vi "MainGUI.vi"() -> ()   [LabVIEW 2018]
uses:
  General/Controls/ScanType.ctl
  General/Controls/Vibratome Parameters.ctl
  General/Controls/Imaging Parameters.ctl
  General/Controls/Scan Direction.ctl
  General/type defines/Alazar parameters.ctl
  Hardware Mfg/AlazarTech SDK/Controls/General Trigger Settings.ctl
  Hardware Mfg/AlazarTech SDK/Controls/Trigger Engine Controls.ctl
  Hardware Mfg/AlazarTech SDK/Controls/Clock Controls.ctl
  Hardware Mfg/AlazarTech SDK/Controls/Alazar Device ID.ctl
  Hardware Mfg/AlazarTech SDK/Controls/Channel Input Controls.ctl
  Hardware Mfg/AlazarTech SDK/Controls/Alazar Acquisition Settings.ctl
  General/Controls/Control cluster.ctl
  General/type defines/file type.ctl
  General/Controls/Optical Parameters.ctl
  General/Controls/Translation Stage Parameters.ctl
  Hardware Mfg/Thorlabs Translation Stages/Controls/Translation Stage Cluster.ctl
  General/Controls/Translation Stage Types.ctl
  General/Controls/Queue Manager Actions.ctl
  General/Controls/MessagePacket.ctl
  General/Controls/QueueNames.ctl
  General/Controls/FGV Actions.ctl
  General/Controls/System Parameters.ctl
  Hardware Mfg/AlazarTech SDK/Controls/Alazar Engine Actions.ctl
  Hardware Mfg/Main Scan Processor Status.vi
  Hardware Mfg/Axsun Laser/Axsun action.ctl
panel:
  in  "Status":string
  in  "Quit":bool
  in  "Acquire":bool
  in  "Control Panel":T1(tab)
  in  "Optical Parameters":T2={"Obj. Focal Length [mm]"=45.0, "Scan Lens EFL[mm]"=59.5, "Tube Lens EFL[mm]"=205.0, "Galvo V Range (+/-)"=10.0, "Galvo Max Half Angle [Deg]"=19.0, "Max Galvo Range[%]"=0.0}
  in  "Galvo HW Parameters":T3={"Analog Out Channel"="GalvoCtrl/ao0,GalvoCtrl/ao1", "Min Voltage"=-10.0, "Max Voltage"=10.0, "Pixel Clock Source"="/GalvoCtrl/PFI0", "Sample Rate"=1000.0, "Line Clock Out Ch"="GalvoCtrl/port0/line0"}
  in  "Imaging Parameter":T4={"Raster Scan Direction"=enum."Uni Directional", "Pixel Dwell Time [Clock Cycles]"=1, "Flyback Time [Clock Cycles]"=200, "XY Center [um]"={"X"=1.0, "Y"=1.0}, "Pixel Step Size [um]"=2.5, "XY Image Size"=enum."2048 x 2048", "Custom"=FALSE, "Custom Size"={"X"=1, "Y"=1}, "Line Averages"=1} {"Line Averages" min=1 max=30 step=1; "Flyback Time [Clock Cycles]" max=1000 step=1; "Pixel Step Size [um]" min=0.0 max=10.0 step=0.01; "Custom Size"."Y" min=1 max=30 step=1; "Custom Size"."X" min=1 max=30 step=1; "XY Center [um]"."Y" min=1.0 max=30.0 step=1.0; "XY Center [um]"."X" min=1.0 max=30.0 step=1.0; "Pixel Dwell Time [Clock Cycles]" max=10 step=1}
  in  "Scan Type":T6
  in  "Alazar parameters":T7={"Trigger Settings"={"General Trigger Settings"={"Trigger Operation"=0, "Coupling ID"=2, "Range ID"=2, "Delay"=0, "Timeout Ticks"=0, "Mode"=1, "Parameter"=1}, "Trigger Engine 1"={"Trigger Engine"=0, "Source"=2, "Slope"=1, "Level"=140}, "Trigger Engine 2"={"Trigger Engine"=1, "Source"=3, "Slope"=1, "Level"=140}}, "Capture Clock"={"Sample Rate"=100, "Decimation"=0, "Source"=2, "Edge"=0}, "Device ID"={"System ID"=1, "Board ID"=1}, "Ch A Input Control"={"Channel"=1, "Coupling"=2, "Range"=10, "Impedance"=2}, "Ch B Input Control"={"Channel"=2, "Coupling"=2, "Range"=10, "Impedance"=2}, "Acq Settings"={"Window Type"=1, "Record Length"=1440, "Footer"=0, "Output Format"=10, "Offset"=0, "Records Per Buffer"=2048, "Samples per record"=2048, "Records Count (Records/Acq)"=2147483647}, "Cluster"={"FFT value magnification"=1000.0, "max queue size (-1, unlimited)"=-1, "File Type"=enum."Tiff", "file path"=path "C:/Users/BoasLab/Documents/Data/Alazar data/B-line/data/test.tif", "#A-lines to save"=2048, "#Z pixels to save"=2048, "ImageDescription"="", "Convert to U16?"=FALSE}} {"Cluster"."FFT value magnification" min=0.0 max=10000.0 step=0.001 format="%.4f"; "Acq Settings"."Window Type" items=["DSP_WINDOW_NONE", "DSP_WINDOW_HANNING", "DSP_WINDOW_HAMMING", "DSP_WINDOW_BLACKMAN", "DSP_WINDOW_BLACKMAN_HARRIS", "DSP_WINDOW_BARTLETT"]; "Acq Settings"."Footer" items=["FOOTER_NONE", "FOOTER_NPT"]; "Acq Settings"."Output Format" items=["FLOAT_AMP2"=10, "FLOAT_LOG"=11]; "Ch B Input Control"."Channel" items=["A"=1, "B"=2, "C"=4, "D"=8]; "Ch B Input Control"."Coupling" items=["AC"=1, "DC"=2]; "Ch B Input Control"."Range" items=["20 mV"=1, "40 mV"=2, "50 mV"=3, "80 mV"=4, "100 mV"=5, "200 mV"=6, "400 mV"=7, "500 mV"=8, "800 mV"=9, "1 V"=10, "1.25 V"=33, "2 V"=11, "4 V"=12, "5 V"=13, "8 V"=14, "10 V"=15, "20 V"=16]; "Ch B Input Control"."Impedance" items=["1 MOhm"=1, "50 Ohm"=2, ""=0]; "Ch A Input Control"."Channel" items=["A"=1, "B"=2, "C"=4, "D"=8]; "Ch A Input Control"."Coupling" items=["AC"=1, "DC"=2]; "Ch A Input Control"."Range" items=["20 mV"=1, "40 mV"=2, "50 mV"=3, "80 mV"=4, "100 mV"=5, "200 mV"=6, "400 mV"=7, "500 mV"=8, "800 mV"=9, "1 V"=10, "1.25 V"=33, "2 V"=11, "4 V"=12, "5 V"=13, "8 V"=14, "10 V"=15, "20 V"=16]; "Ch A Input Control"."Impedance" items=["1 MOhm"=1, "50 Ohm"=2, ""=0]; "Capture Clock"."Edge" items=["Rising", "Falling"]; "Capture Clock"."Source" items=["Internal"=1, "Fast External"=2, "Medium External"=3, "Slow External"=4, "External AC"=5, "External DC"=6, "External 10MHz"=7]; "Trigger Settings"."General Trigger Settings"."Trigger Operation" items=["J", "K", "J OR K", "J AND K", "J XOR K", "J AND NOT K", "NOT J AND K"]; "Trigger Settings"."General Trigger Settings"."Coupling ID" items=["AC"=1, "DC"=2]; "Trigger Settings"."General Trigger Settings"."Range ID" items=["5 V", "1 V", "TTL"]; "Trigger Settings"."Trigger Engine 1"."Trigger Engine" items=["J", "K"]; "Trigger Settings"."Trigger Engine 1"."Source" items=["A", "B", "External", "Disable", "C", "D"]; "Trigger Settings"."Trigger Engine 1"."Slope" items=["Positive"=1, "Negative"=2]; "Trigger Settings"."Trigger Engine 2"."Trigger Engine" items=["J", "K"]; "Trigger Settings"."Trigger Engine 2"."Source" items=["A", "B", "External", "Disable", "C", "D"]; "Trigger Settings"."Trigger Engine 2"."Slope" items=["Positive"=1, "Negative"=2]}
  in  "Vibratome":T16={"Z Bottom [mm]"=0.0, "Pre Cut Dwell [s]"=0.0, "Blade Frequency [RPM]"=0, "Slice Speed [mm/s]"=0.0, "Post Cut Dwell [s]"=0.0, "Ramp Time [s]"=0.0, "Start X [mm]"=0.0, "Start Y [mm]"=0.0, "Slice Length [mm]"=0.0, "Slice Axis"=enum."X Axis", "Controller VISA Ref"="COM4"}
  in  "Mosaic Paramter":T17
  in  "Center Galvos":bool
  in  "path":path=path "C:/Users/BOAS-USER/Documents/Data/0507/human"
  out "time for pre-process":dbl
  out "Error Out":errorcluster
  in  "#pixels to save":i32=200
  in  "start pixel":i32
  in  "Save":bool
  out "elements in display queue":i32
  out "# elements in save queue":i32
  in  "display pixels":i32=500
  in  "FOV: #A-lines":i32=2048
  in  "Init":bool
  in  "Channel":u32(ring)=1 items=["A"=1, "B"=2, "A + B"=3, "C"=4, "A + C"=5, "A + B"=6, "D"=8, "A + D"=9, "B + D"=10, "C + D"=12, "A + B + C + D"=15]
  out "#C-lines":i32=1
  out "# elements in data queue":i32
  in  "Start pixel for display":i32=1
  out "Current Position":cluster{"X":dbl, "Y":dbl}
  in  "Table Stages":T18={"X Stage"={"Position"=0.0, "Is.Enabled?"=FALSE, "Is.Connected?"=FALSE, "Device SN"="45876539", "AccelerationMaximum"=20.0, "VelocityMaximum"=20.0, "Acceleration"=10.0, "Velocity"=10.0, "waitTimeout (ms)"=1000, "Model"=enum."Thorlabs LTS", "Is.Homed?"=FALSE}, "Y Stage"={"Position"=0.0, "Is.Enabled?"=FALSE, "Is.Connected?"=FALSE, "Device SN"="45876539", "AccelerationMaximum"=0.0, "VelocityMaximum"=0.0, "Acceleration"=0.0, "Velocity"=0.0, "waitTimeout (ms)"=0, "Model"=enum."None", "Is.Homed?"=FALSE}, "Z Stage"={"Position"=0.0, "Is.Enabled?"=FALSE, "Is.Connected?"=FALSE, "Device SN"="49876924", "AccelerationMaximum"=8.0, "VelocityMaximum"=3.0, "Acceleration"=4.0, "Velocity"=2.0, "waitTimeout (ms)"=1000, "Model"=enum."Thorlabs MLJ", "Is.Homed?"=FALSE}}
  out "Image":T21(plugin-control)
  out "Control Class ID":u32[](array[numeric])
  out "Label Name":string[][](array[string])
  # "Image Settings"
  # "Optical Settings"
  # "X"
  # "X"
  # "Vibratome Settings"
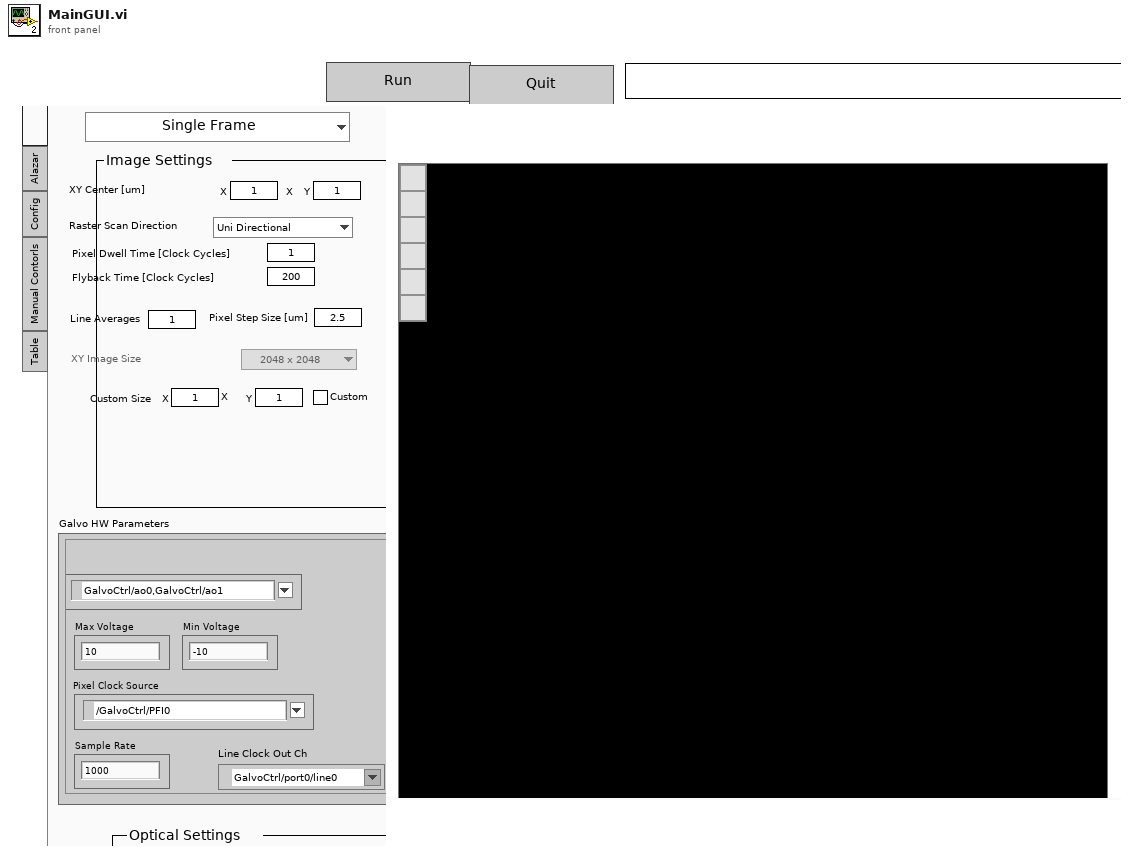
[diagram p1: front panel]
types:
  T1 = enum32{"Galvo", "Alazar", "Config", "Manual Contorls", "Table"}
  T2 = typedef "Optical Parameters.ctl" = cluster{"Obj. Focal Length [mm]":dbl, "Scan Lens EFL[mm]":dbl, "Tube Lens EFL[mm]":dbl, "Galvo V Range (+/-)":dbl, "Galvo Max Half Angle [Deg]":dbl, "Max Galvo Range[%]":dbl}
  T3 = cluster{"Analog Out Channel":tag, "Min Voltage":dbl, "Max Voltage":dbl, "Pixel Clock Source":tag, "Sample Rate":dbl, "Line Clock Out Ch":tag}
  T4 = typedef "Imaging Parameters.ctl" = cluster{"Raster Scan Direction":T5, "Pixel Dwell Time [Clock Cycles]":u16, "Flyback Time [Clock Cycles]":u16, "XY Center [um]":cluster{"X":dbl, "Y":dbl}, "Pixel Step Size [um]":dbl, "XY Image Size":enum16{"32 x 32", "64 x 64", "128 x 128", "256 x 256", "512 x 512", "1024 x 1024", "2048 x 2048"}, "Custom":bool, "Custom Size":cluster{"X":u16, "Y":u16}, "Line Averages":u8}
  T5 = typedef "Scan Direction.ctl" = enum16{"Uni Directional", "Bi Directional", "None"}
  T6 = typedef "ScanType.ctl" = enum16{"Single Frame", "Continuous Frame", "ROI Line", "Vibratome", "Mosaic", "Mosaic + Slice"}
  T7 = typedef "Alazar parameters.ctl" = cluster{"Trigger Settings":cluster{"General Trigger Settings":T8, "Trigger Engine 1":T9, "Trigger Engine 2":T9}, "Capture Clock":T10, "Device ID":T11, "Ch A Input Control":T12, "Ch B Input Control":T12, "Acq Settings":T13, "Cluster":T14}
  T8 = typedef "General Trigger Settings.ctl" = cluster{"Trigger Operation":u32, "Coupling ID":u32, "Range ID":u32, "Delay":u32, "Timeout Ticks":u32, "Mode":u32, "Parameter":u32}
  T9 = typedef "Trigger Engine Controls.ctl" = cluster{"Trigger Engine":u32, "Source":u32, "Slope":u32, "Level":u32}
  T10 = typedef "Clock Controls.ctl" = cluster{"Sample Rate":u32, "Decimation":u32, "Source":u32, "Edge":u32}
  T11 = typedef "Alazar Device ID.ctl" = cluster{"System ID":u32, "Board ID":u32}
  T12 = typedef "Channel Input Controls.ctl" = cluster{"Channel":u8, "Coupling":u32, "Range":u32, "Impedance":u32}
  T13 = typedef "Alazar Acquisition Settings.ctl" = cluster{"Window Type":u32, "Record Length":u32, "Footer":u32, "Output Format":u32, "Offset":u32, "Records Per Buffer":u32, "Samples per record":u32, "Records Count (Records/Acq)":u32}
  T14 = typedef "Control cluster.ctl" = cluster{"FFT value magnification":dbl, "max queue size (-1, unlimited)":i32, "File Type":T15, "file path":path, "#A-lines to save":u32, "#Z pixels to save":u32, "ImageDescription":string, "Convert to U16?":bool}
  T15 = typedef "file type.ctl" = enum16{"text", "Tiff", "binary"}
  T16 = typedef "Vibratome Parameters.ctl" = cluster{"Z Bottom [mm]":dbl, "Pre Cut Dwell [s]":dbl, "Blade Frequency [RPM]":u16, "Slice Speed [mm/s]":dbl, "Post Cut Dwell [s]":dbl, "Ramp Time [s]":dbl, "Start X [mm]":dbl, "Start Y [mm]":dbl, "Slice Length [mm]":dbl, "Slice Axis":enum16{"X Axis", "Y Axis", "Z Axis"}, "Controller VISA Ref":refnum<visa-resource-name>}
  T17 = cluster{"X Axis":cluster{"Start [mm]":dbl, "Steps [pts]":u16, "End [mm]":dbl}, "Y Axis":cluster{"Start [mm]":dbl, "Steps [pts]":u16, "End [mm]":dbl}, "Scan Pattern":enum16{"Uni-directional", "Bi-Directional", "Spiral Out", "Spiral In"}, "Overlap Options":cluster{"Overlap Type":enum16{"No Overlap", "X Only", "Y Only", "X and Y"}, "Percent Overlap":u8, "Justify":enum16{"Start", "Center", "End"}}}
  T18 = typedef "Translation Stage Parameters.ctl" = cluster{"X Stage":T19, "Y Stage":T19, "Z Stage":T19}
  T19 = typedef "Translation Stage Cluster.ctl" = cluster{"Position":dbl, "Is.Enabled?":bool, "Is.Connected?":bool, "Device SN":string, "AccelerationMaximum":dbl, "VelocityMaximum":dbl, "Acceleration":dbl, "Velocity":dbl, "waitTimeout (ms)":i32, "Model":T20, "Is.Homed?":bool}
  T20 = typedef "Translation Stage Types.ctl" = enum16{"None", "Thorlabs LTS", "Thorlabs MLJ"}
  T21 = typedef "IMAQ Image.ctl" = refnum<image>
  T22 = typedef "QueueNames.ctl" = enum16{"Main GUI", "Main Scan Processor", "Main Processing", "Main Saving", "Main Display", "Main Table Stage GUI", "Main Table Stage Proc.", "Scan Engine", "Vibratome GUI", "Vibratome Processor", "Slice Engine"}
  T23 = typedef "Queue Manager Actions.ctl" = enum16{"Init", "Enqueue", "Enqueue All", "Preview Queue", "Dequeue", "Get Status", "Flush Queue", "Flush All Queues", "Release All Queues", "Release Queue", "Enqueue at Opposite End"}
  T24 = typedef "MessagePacket.ctl" = cluster{"Message":string, "Parameter":variant}
  T25 = typedef "Image Type" = u32
  T26 = typedef "Axsun action.ctl" = enum16{"GetSystemStatus", "Clock delay", "GetLaserOnTime", "GetWaveLengthAtSweptTrigger", "Source current ON", "GetSerialNum", "GetControlVersion", "Laser ON", "Laser OFF", "Source current OFF", "Get laser handle", "Start Network Control Interface", "stop", "Create handle"}
  T27 = typedef "FGV Actions.ctl" = enum16{"Init", "Set", "Get", "Clear"}
  T28 = typedef "Alazar Engine Actions.ctl" = enum16{"Init", "Config Clock", "Config Ch", "Config Trig", "Config Non-FFT Acq.", "Non-FFT Acquire", "Load background from Non-FFT buffer", "enable background subtrac", "disable background subtrac", "load background from file", "load background from elsewhere", "start acquire", "background subtraction", "Config Acq.", "Acquire", "UnInit"}
  T29 = enum16{"Set Configuration", "Get Configuration", "Enable Motor", "Disable Motor", "Get Status", "Open Session", "Close Session", "Set Limits", "Get Limits"}
  T30 = typedef "System Parameters.ctl" = cluster{"Optical Parameters":T2, "Vibratome":T16, "Table Stages":T18, "Imaging Parameter":T4, "Galvo HW Parameters":cluster{"Analog Out Channel":tag, "Min Voltage":dbl, "Max Voltage":dbl, "Pixel Clock Source":tag, "Sample Rate":dbl, "Line Clock Out Ch":tag}, "Alazar parameters":T7, "Mosaic Paramter":cluster{"X Axis":cluster{"Start [mm]":dbl, "Steps [pts]":u16, "End [mm]":dbl}, "Y Axis":cluster{"Start [mm]":dbl, "Steps [pts]":u16, "End [mm]":dbl}, "Scan Pattern":enum16{"Uni-directional", "Bi-Directional", "Spiral Out", "Spiral In"}, "Overlap Options":cluster{"Overlap Type":enum16{"No Overlap", "X Only", "Y Only", "X and Y"}, "Percent Overlap":u8, "Justify":enum16{"Start", "Center", "End"}}}}
  T31 = enum16{"32 x 32", "64 x 64", "128 x 128", "256 x 256", "512 x 512", "1024 x 1024", "2048 x 2048"}
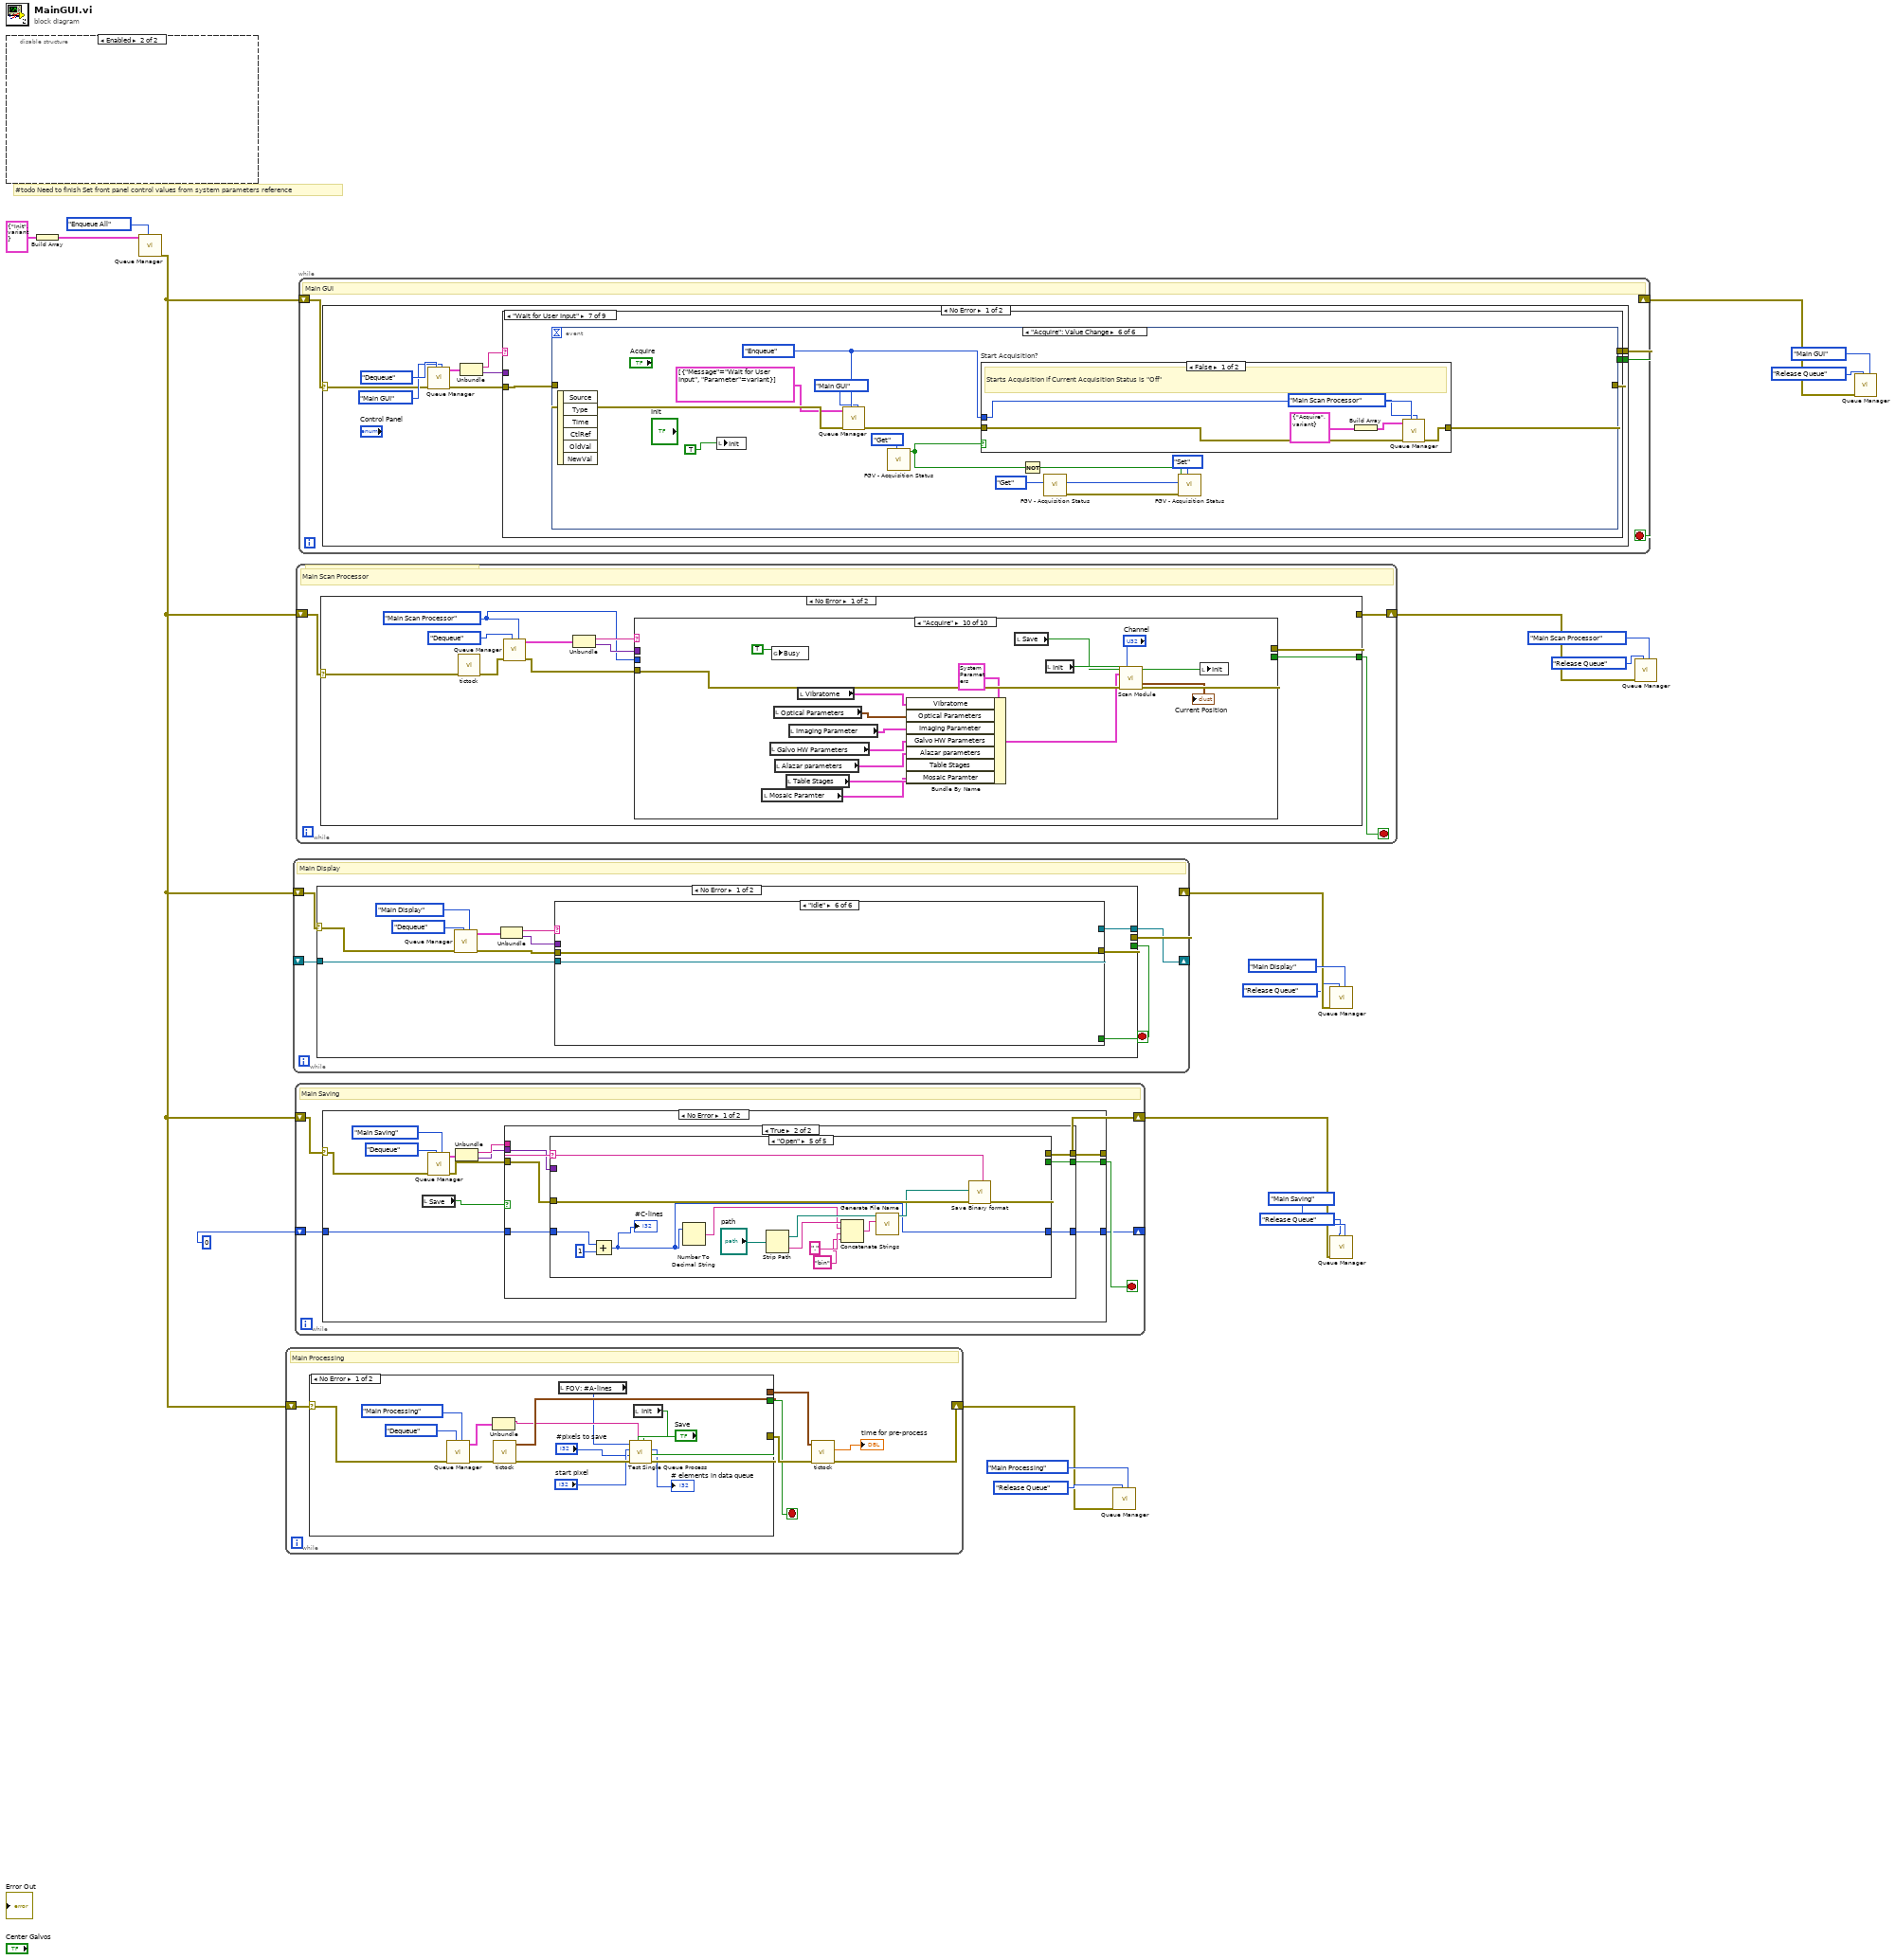
[diagram p0: block diagram]
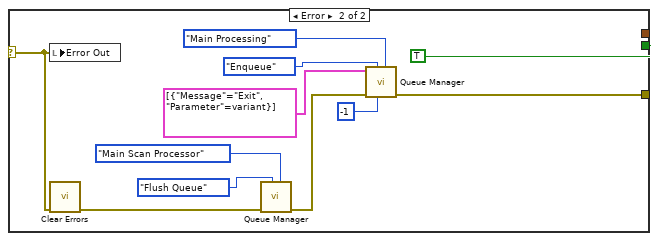
[diagram p2: hidden frame]
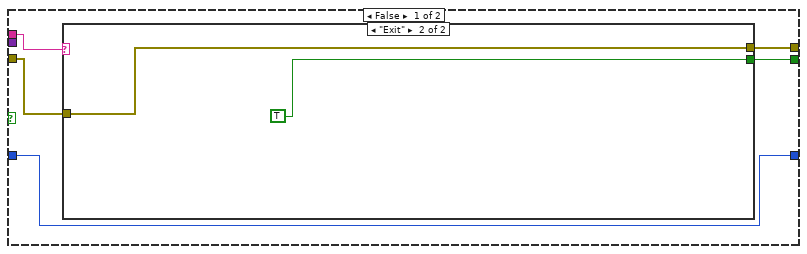
[diagram p3: hidden frame]
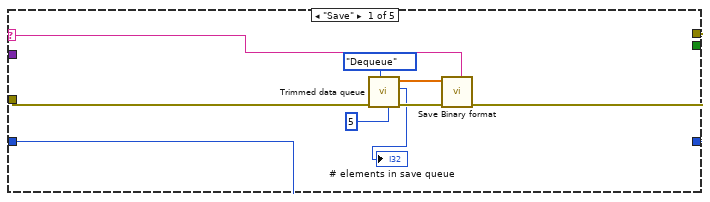
[diagram p5: hidden frame]
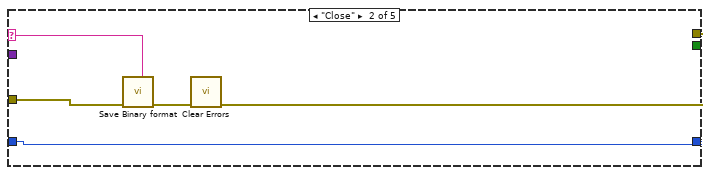
[diagram p6: hidden frame]
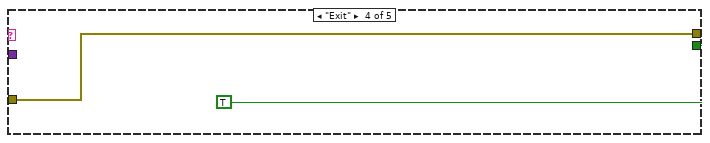
[diagram p8: hidden frame]
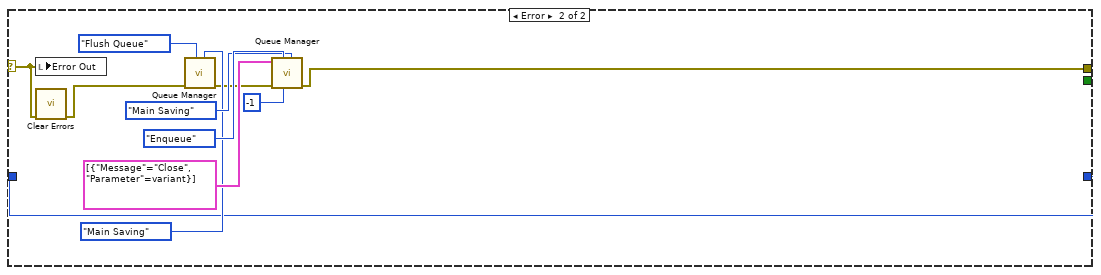
[diagram p9: hidden frame]
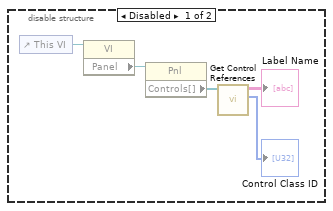
[diagram p10: hidden frame]
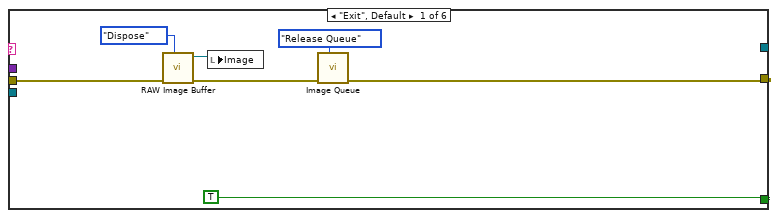
[diagram p11: hidden frame]
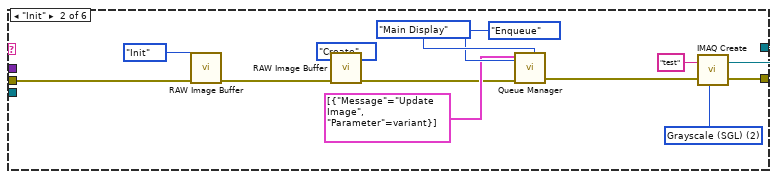
[diagram p12: hidden frame]
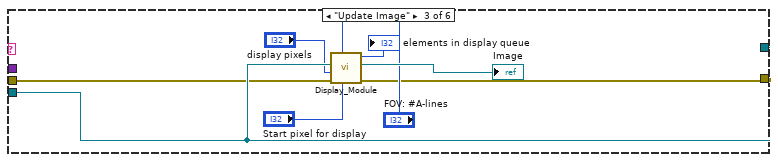
[diagram p13: hidden frame]
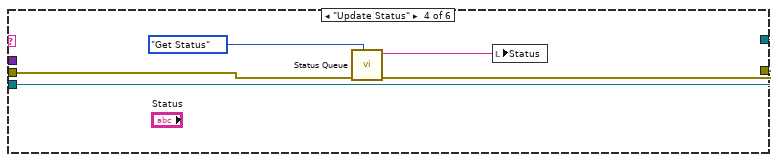
[diagram p14: hidden frame]
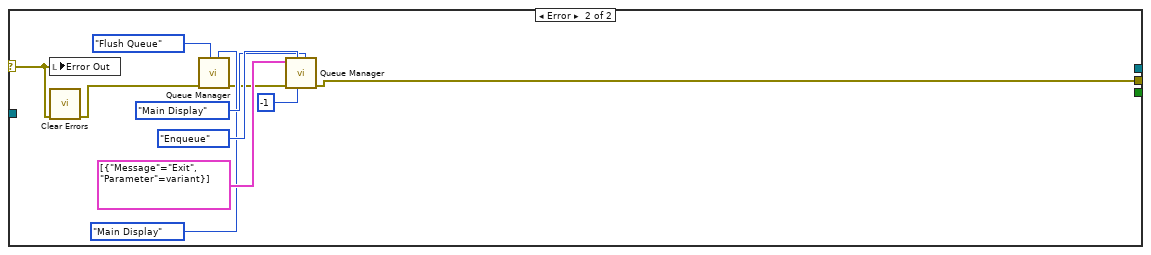
[diagram p16: hidden frame]
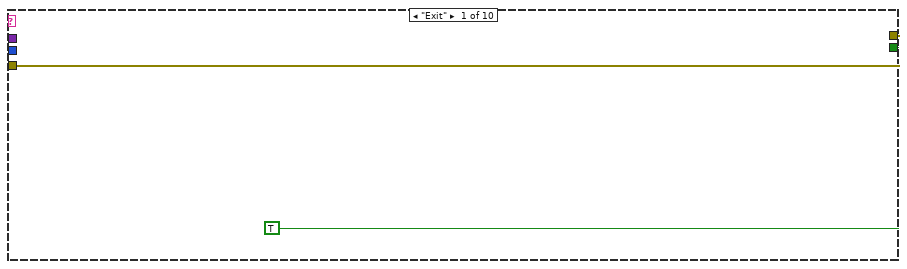
[diagram p17: hidden frame]
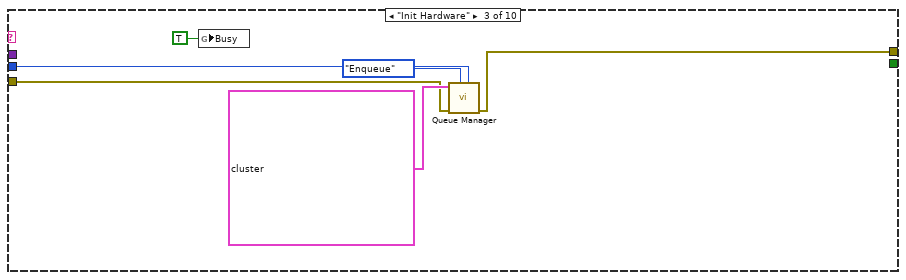
[diagram p19: hidden frame]
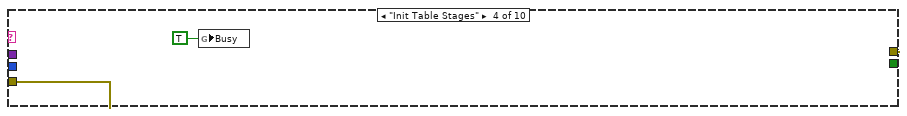
[diagram p20: hidden frame]
diagram:
  # "#todo Add indicator to show connected HW"
  # "#todo Need to finish Set front panel control values from system parameters reference"
  n1 = disable-structure shown="Enabled" {
    frame Disabled {
      n2 = control-ref of="This VI"() -> (w25:refnum<vi>)
      n3 = property class="VI"(reference=w25) -> ("Panel"=w24:refnum<vi>)  [unwired: 1 in, 2 out]
      n4 = property class="Pnl"(reference=w24) -> ("Controls[]"=w23:refnum<vi>[])  [unwired: 1 in, 2 out]
      n5 = call "Get Control References.vi"("Control References"=w23) -> ("Control Class ID"=→"Control Class ID":u32[], "Label Name"=→"Label Name":string[][])  [unwired: 8 in, 1 out]
    }
    frame Enabled {
    }
  }
  n6 = Build Array(T24 {"Message"="Init", "Parameter"=variant} ("Message Packet [In]")) -> (w18:T24[])
  n7 = call "Queue Manager.vi"("Action"=Queue_Manager_Actions."Enqueue All", "Message Packet Array"=w18) -> ("Error Out"=w2:errorcluster)  [unwired: 5 in, 4 out]
  n8 = while "Main Data Processing" {
    shift-right: [w30] -> w3
    shift-left: w2 -> [w28]
    stop <- w26 stop-if-true
    # "Main Processing"
    n9 = case shown="No Error" w28 {
      selector: w28 -> [w42 w54]
      tunnel: [w40 w53] -> w31
      tunnel: [w43 _] -> w29
      tunnel: [w39 TRUE ("Exit?")] -> w26
      frame No Error {
        n10 = call "Queue Manager.vi"("Queue Name"=QueueNames."Main Processing", "Action"=Queue_Manager_Actions."Dequeue", "Error In"=w42) -> ("Error Out"=w44:errorcluster, "Message Packet [Out]"=w45:T24)  [unwired: 4 in, 3 out]
        n11 = Unbundle(w45) -> ("Message"=w37:string)  [unwired: 1 out]
        n12 = call "tictock.vi"("error in (no error)"=w44) -> ("error out"=w41:errorcluster, "seconds since 1Jan1904"=w43:timestamp)  [unwired: 8 in, 1 out]
        n13 = local read "FOV: #A-lines"() -> (w36:i32)
        n14 = local read "Init"() -> (w32:bool)
        n15 = call "Test Single Queue Process.vi"("Init?"=w32, "Action"=w37, "Save"="Save", "error in"=w41, "#pixels to save"="#pixels to save", "start pixel"="start pixel", "#A-lines per B-line"=w36) -> ("Error Out"=w40:errorcluster, "Exit?"=w39:bool, "# elements in data queue"=→"# elements in data queue":i32)  [unwired: 2 in]
      }
      frame Error {
        n16 = local write "Error Out"(w54) -> ()
        n17 = call <vilib>:"Clear Errors.vi"("error in (no error)"=w54) -> ("error out"=w50:errorcluster)  [unwired: 5 in, 1 out]
        n18 = call "Queue Manager.vi"("Queue Name"=QueueNames."Main Scan Processor", "Action"=Queue_Manager_Actions."Flush Queue", "Error In"=w50) -> ("Error Out"=w49:errorcluster)  [unwired: 4 in, 4 out]
        n19 = call "Queue Manager.vi"("Queue Name"=QueueNames."Main Processing", "timeout in ms (-1)"=-1, "Action"=Queue_Manager_Actions."Enqueue", "Error In"=w49, "Message Packet Array"=T24[] [{"Message"="Exit", "Parameter"=variant}] ("Message Packet [In]")) -> ("Error Out"=w53:errorcluster)  [unwired: 2 in, 4 out]
      }
    }
    n20 = call "tictock.vi"("error in (no error)"=w31, "seconds since 1Jan1904 2"=w29) -> ("error out"=w30:errorcluster, "Numeric"=→"time for pre-process":dbl)  [unwired: 7 in, 1 out]
  }
  n21 = while {
    shift-right: [w63] -> w10
    shift-left: w2 -> [w59]
    shift-right: [w61] -> _
    shift-left: _ -> [w60]
    stop <- w62 stop-if-true
    # "Main Display"
    n22 = case shown="No Error" w59 {
      selector: w59 -> [w64 w117]
      tunnel: [w68 w116] -> w63
      tunnel: [w67 _] -> w62
      tunnel: [w66 _] -> w61
      tunnel: w60 -> [w65 _]
      frame No Error {
        n23 = call "Queue Manager.vi"("Queue Name"=QueueNames."Main Display", "Action"=Queue_Manager_Actions."Dequeue", "Error In"=w64) -> ("Error Out"=w72:errorcluster, "Message Packet [Out]"=w71:T24)  [unwired: 4 in, 3 out]
        n24 = Unbundle(w71) -> ("Message"=w70:string, "Parameter"=w69:variant)
        n25 = case shown="\"Idle\"" w70 {
          tunnel: w72 -> [w79 w94 w95 w107 w109 w111]
          tunnel: w69 -> [_ _ _ _ _ _]
          tunnel: [w77 w82 w96 w106 w109 w111] -> w68
          tunnel: [TRUE _ _ _ _ _] -> w67
          tunnel: [_ w88 w102 w103 w108 w110] -> w66
          tunnel: w65 -> [_ _ w102 w103 w108 w110]
          frame "Exit", Default {
            n26 = call "RAW Image Buffer.vi"("Actions"=enum16{"Init", "Create", "Get", "Dispose"}."Dispose", "Error In"=w79) -> ("Error Out"=w78:errorcluster, "Image Out"=w75:T21)  [unwired: 8 in]
            n27 = local write "Image"(w75) -> ()
            n28 = call "Image Queue.vi"("Action"=Queue_Manager_Actions."Release Queue", "Error In"=w78) -> ("Error Out"=w77:errorcluster)  [unwired: 8 in, 1 out]
          }
          frame "Init" {
            w89 = T25 2 items=["Grayscale (U8)", "Grayscale (I16)", "Grayscale (SGL)", "Complex (CSG)", "RGB (U32)", "HSL (U32)", "RGB (U64)", "Grayscale (U16)"] ("Image Type")
            n29 = call "RAW Image Buffer.vi"("Actions"=enum16{"Init", "Create", "Get", "Dispose"}."Init", "Error In"=w94) -> ("Error Out"=w93:errorcluster)  [unwired: 8 in, 1 out]
            n30 = call "RAW Image Buffer.vi"("Actions"=enum16{"Init", "Create", "Get", "Dispose"}."Create", "Error In"=w93) -> ("Error Out"=w84:errorcluster)  [unwired: 8 in, 1 out]
            n31 = call "Queue Manager.vi"("Queue Name"=QueueNames."Main Display", "Action"=Queue_Manager_Actions."Enqueue", "Error In"=w84, "Message Packet Array"=T24[] [{"Message"="Update Image", "Parameter"=variant}]) -> ("Error Out"=w83:errorcluster)  [unwired: 3 in, 4 out]
            n32 = call "IMAQ Create"("Image Name"="test", "Image Type"=w89, "error in (no error)"=w83) -> ("New Image"=w88:T21, "error out"=w82:errorcluster)  [unwired: 2 in]
          }
          frame "Update Image" {
            n33 = call "Display_Module.vi"("Start pixel for display"="Start pixel for display", "FOV: #A-lines"="FOV: #A-lines", "error in"=w95, "Total pixels to display"="display pixels", "Source in"=w102) -> ("error out"=w96:errorcluster, "Image"=→"Image":T21, "elements in display queue"=→"elements in display queue":i32)  [unwired: 4 in]
          }
          frame "Update Status" {
            n34 = call "Status Queue.vi"("Action"=Queue_Manager_Actions."Get Status", "Error In"=w107) -> ("Error Out"=w106:errorcluster, "Status Message [Out]"=w104:string)  [unwired: 8 in]
            n35 = local write "Status"(w104) -> ()
          }
          frame "Update Line Profile" {
          }
          frame "Idle" {
          }
        }
      }
      frame Error {
        n36 = local write "Error Out"(w117) -> ()
        n37 = call <vilib>:"Clear Errors.vi"("error in (no error)"=w117) -> ("error out"=w113:errorcluster)  [unwired: 5 in, 1 out]
        n38 = call "Queue Manager.vi"("Queue Name"=QueueNames."Main Display", "Action"=Queue_Manager_Actions."Flush Queue", "Error In"=w113) -> ("Error Out"=w112:errorcluster)  [unwired: 4 in, 4 out]
        n39 = call "Queue Manager.vi"("Queue Name"=QueueNames."Main Display", "timeout in ms (-1)"=-1, "Action"=Queue_Manager_Actions."Enqueue", "Error In"=w112, "Message Packet Array"=T24[] [{"Message"="Exit", "Parameter"=variant}] ("Message Packet [In]")) -> ("Error Out"=w116:errorcluster)  [unwired: 2 in, 4 out]
      }
    }
  }
  n40 = while {
    shift-right: [w126] -> w6
    shift-left: w2 -> [w124]
    shift-right: [w123] -> _
    shift-left: 0 -> [w122]
    stop <- w125 stop-if-true
    # "Main Saving"
    n41 = case shown="No Error" w124 {
      selector: w124 -> [w136 w192]
      tunnel: [w138 w191] -> w126
      tunnel: [w137 _] -> w125
      tunnel: [w135 w186] -> w123
      tunnel: w122 -> [w134 w186]
      frame No Error {
        n42 = local read "Save"() -> (w133:bool)
        n43 = call "Queue Manager.vi"("Queue Name"=QueueNames."Main Saving", "Action"=Queue_Manager_Actions."Dequeue", "Error In"=w136) -> ("Error Out"=w127:errorcluster, "Message Packet [Out]"=w132:T24)  [unwired: 4 in, 3 out]
        n44 = Unbundle(w132) -> ("Message"=w129:string, "Parameter"=w128:variant)
        n45 = case shown="True" w133 {
          tunnel: [w142 w153] -> w138
          tunnel: [w139 w152] -> w137
          tunnel: [w140 w151] -> w135
          tunnel: w134 -> [w140 w150]
          tunnel: w129 -> [w141 w149]
          tunnel: w128 -> [_ w148]
          tunnel: w127 -> [w143 w147]
          frame False {
            n46 = case shown="\"Exit\"" w141 {
              tunnel: [w144 w145] -> w142
              tunnel: w143 -> [w144 w145]
              tunnel: [_ TRUE] -> w139
              frame "Init", Default {
              }
              frame "Exit" {
              }
            }
          }
          frame True {
            n47 = case shown="\"Open\"" w149 {
              selector: w149 -> [w161 w166 _ _ w184]
              tunnel: [w159 w163 w169 w170 w175] -> w153
              tunnel: w148 -> [_ _ _ _ _]
              tunnel: w147 -> [w162 w167 w169 w170 w185]
              tunnel: [_ _ _ TRUE _] -> w152
              tunnel: [w160 w164 w168 _ w173] -> w151
              tunnel: w150 -> [w160 w164 w168 _ w172]
              frame "Save" {
                n48 = call "Trimmed data queue.vi"("timeout in ms (-1)"=5, "Action"=Queue_Manager_Actions."Dequeue", "error in (no error)"=w162) -> ("error out"=w157:errorcluster, "# elements in queue"=→"# elements in save queue":i32, "data out"=w158:sgl[])  [unwired: 5 in, 1 out]
                n49 = call "Save Binary format.vi"("action"=w161, "error in"=w157, "data in"=w158) -> ("error out"=w159:errorcluster)  [unwired: 8 in]
              }
              frame "Close" {
                n50 = call "Save Binary format.vi"("action"=w166, "error in"=w167) -> ("error out"=w165:errorcluster)  [unwired: 9 in]
                n51 = call <vilib>:"Clear Errors.vi"("error in (no error)"=w165) -> ("error out"=w163:errorcluster)  [unwired: 5 in, 1 out]
              }
              frame "Init", Default {
              }
              frame "Exit" {
              }
              frame "Open" {
                n52 = Add(x=w172, y=1) -> (x+y=w173:i32)
                "#C-lines" <- w173
                n53 = Number To Decimal String(number=w173) -> (decimal integer string=w178:string)  [unwired: 1 in]
                n54 = Strip Path(path="path") -> (stripped path=w182:path, name=w183:string)
                n55 = Concatenate Strings(w183, w178, "." ("string"), "bin" ("string")) -> (w181:string)
                n56 = call "Generate File Name.vi"("name or relative path"=w181, "base path"=w182) -> ("appended path"=w180:path)  [unwired: 9 in]
                n57 = call "Save Binary format.vi"("action"=w184, "error in"=w185, "file path (use dialog)"=w180) -> ("error out"=w175:errorcluster)  [unwired: 8 in]
              }
            }
          }
        }
      }
      frame Error {
        n58 = local write "Error Out"(w192) -> ()
        n59 = call <vilib>:"Clear Errors.vi"("error in (no error)"=w192) -> ("error out"=w188:errorcluster)  [unwired: 5 in, 1 out]
        n60 = call "Queue Manager.vi"("Queue Name"=QueueNames."Main Saving", "Action"=Queue_Manager_Actions."Flush Queue", "Error In"=w188) -> ("Error Out"=w187:errorcluster)  [unwired: 4 in, 4 out]
        n61 = call "Queue Manager.vi"("Queue Name"=QueueNames."Main Saving", "timeout in ms (-1)"=-1, "Action"=Queue_Manager_Actions."Enqueue", "Error In"=w187, "Message Packet Array"=T24[] [{"Message"="Close", "Parameter"=variant}] ("Message Packet [In]")) -> ("Error Out"=w191:errorcluster)  [unwired: 2 in, 4 out]
      }
    }
  }
  n62 = while {
    shift-right: [w198] -> w12
    shift-left: w2 -> [w197]
    stop <- w199 stop-if-true
    # "Main Scan Processor"
    n63 = case shown="No Error" w197 {
      selector: w197 -> [w202 w284]
      tunnel: [w205 _] -> w199
      tunnel: [w200 w279] -> w198
      frame No Error {
        w204 = QueueNames."Main Scan Processor" ("Queue Name")
        n64 = call "tictock.vi"("error in (no error)"=w202) -> ("error out"=w203:errorcluster)  [unwired: 8 in, 2 out]
        n65 = call "Queue Manager.vi"("Queue Name"=w204, "Action"=Queue_Manager_Actions."Dequeue", "Error In"=w203) -> ("Error Out"=w201:errorcluster, "Message Packet [Out]"=w208:T24)  [unwired: 4 in, 3 out]
        n66 = Unbundle(w208) -> ("Message"=w207:string, "Parameter"=w206:variant)
        n67 = case shown="\"Acquire\"" w207 {
          tunnel: w206 -> [_ _ _ _ _ _ _ _ _ _]
          tunnel: [w210 w212 w218 w219 w221 w223 w242 w246 w256 w273] -> w200
          tunnel: [TRUE _ _ _ _ _ _ _ _ _] -> w205
          tunnel: w204 -> [_ _ w217 _ _ _ _ _ _ _]
          tunnel: w201 -> [w210 w212 w213 w219 w221 w222 w237 w245 w256 w270]
          frame "Exit" {
          }
          frame "Init" {
          }
          frame "Init Hardware" {
            n68 = global write "Main Scan Processor Status.vi" "Busy"(TRUE ("Busy")) -> ()
            n69 = call "Queue Manager.vi"("Queue Name"=w217, "Action"=Queue_Manager_Actions."Enqueue", "Error In"=w213, "Message Packet Array"=T24[] [{"Message"="Init Table Stages", "Parameter"=variant}, {"Message"="Init DAQ", "Parameter"=variant}, {"Message"="Init Vibratome", "Parameter"=variant}, {"Message"="Idle", "Parameter"=variant}, {"Message"="Init Laser", "Parameter"=variant}, {"Message"="Init Alazar", "Parameter"=variant}, {"Message"="Init Table Stages", "Parameter"=variant}]) -> ("Error Out"=w218:errorcluster)  [unwired: 3 in, 4 out]
          }
          frame "Init Table Stages" {
            n70 = global write "Main Scan Processor Status.vi" "Busy"(TRUE ("Busy")) -> ()
          }
          frame "Init DAQ" {
          }
          frame "Init Laser" {
            n71 = disable-structure shown="Disabled" {
              disable-tunnel: w222 -> [w225 _]
              disable-tunnel: [w224 _] -> w223
              frame Disabled {
                n72 = call "Axsun module.vi"("Action"=Axsun_action."Create handle", "error in (no error)"=w225) -> ("error out"=w235:errorcluster)  [unwired: 8 in, 1 out]
                n73 = call "Axsun module.vi"("Action"=Axsun_action."GetControlVersion", "error in (no error)"=w235) -> ("error out"=w234:errorcluster)  [unwired: 8 in, 1 out]
                n74 = call "Axsun module.vi"("Action"=Axsun_action."Start Network Control Interface", "error in (no error)"=w234) -> ("error out"=w233:errorcluster)  [unwired: 8 in, 1 out]
                n75 = call "Axsun module.vi"("Action"=Axsun_action."Get laser handle", "error in (no error)"=w233) -> ("error out"=w232:errorcluster)  [unwired: 8 in, 1 out]
                n76 = call "Axsun module.vi"("Action"=Axsun_action."GetSerialNum", "error in (no error)"=w232) -> ("error out"=w231:errorcluster)  [unwired: 8 in, 1 out]
                n77 = call "Axsun module.vi"("Action"=Axsun_action."GetSystemStatus", "error in (no error)"=w231) -> ("error out"=w224:errorcluster)  [unwired: 8 in, 1 out]
              }
              frame Enabled {
              }
            }
          }
          frame "Init Alazar" {
            n78 = call "System Parameters - FGV.vi"("Actions"=FGV_Actions."Get", "Error In"=w237) -> ("Error Out"=w240:errorcluster, "System Parameters"=w239:T30)  [unwired: 8 in]
            n79 = Unbundle By Name(w239) -> ("Alazar parameters"=w238:T7)
            n80 = Unbundle By Name(w238) -> ("Device ID"=w243:T11)
            n81 = call "AlazarEngine.vi"("Action"=Alazar_Engine_Actions."Init", "error in (no error)"=w240, "Device ID"=w243) -> ("error out"=w242:errorcluster)  [unwired: 6 in, 2 out]
          }
          frame "Init Vibratome" {
            n82 = disable-structure shown="Disabled" {
              disable-tunnel: w245 -> [w252 _]
              disable-tunnel: [w251 _] -> w246
              frame Disabled {
                n83 = call "System Parameters - FGV.vi"("Actions"=FGV_Actions."Get") -> ("System Parameters"=w249:T30)  [unwired: 9 in, 1 out]
                n84 = Unbundle By Name(w249) -> ("Vibratome.Controller VISA Ref"=w248:refnum<visa-resource-name>)
                n85 = call "MCDC3006 Module.vi"("Actions"=T29."Open Session", "Error In"=w252, "VISA resource name"=w248) -> ("Error Out"=w254:errorcluster)  [unwired: 4 in, 4 out]
                n86 = call "MCDC3006 Module.vi"("Actions"=T29."Enable Motor", "Error In"=w254) -> ("Error Out"=w251:errorcluster)  [unwired: 5 in, 4 out]
              }
              frame Enabled {
              }
            }
            n87 = global write "Main Scan Processor Status.vi" "Busy"(TRUE ("Busy")) -> ()
          }
          frame "Idle", Default {
            n88 = global write "Main Scan Processor Status.vi" "Busy"(FALSE ("Busy")) -> ()
          }
          frame "Acquire" {
            n89 = local read "Mosaic Paramter"() -> (w260:T17)
            n90 = local read "Galvo HW Parameters"() -> (w265:T3)
            n91 = global write "Main Scan Processor Status.vi" "Busy"(TRUE ("Busy")) -> ()
            n92 = local read "Optical Parameters"() -> (w267:T2)
            n93 = local read "Alazar parameters"() -> (w264:T7)
            n94 = local read "Table Stages"() -> (w263:T18)
            n95 = local read "Imaging Parameter"() -> (w266:T4)
            n96 = local read "Vibratome"() -> (w268:T16)
            n97 = Bundle By Name(cluster=T30 {"Optical Parameters"={"Obj. Focal Length [mm]"=0.0, "Scan Lens EFL[mm]"=0.0, "Tube Lens EFL[mm]"=0.0, "Galvo V Range (+/-)"=0.0, "Galvo Max Half Angle [Deg]"=0.0, "Max Galvo Range[%]"=0.0}, "Vibratome"={"Z Bottom [mm]"=0.0, "Pre Cut Dwell [s]"=0.0, "Blade Frequency [RPM]"=0, "Slice Speed [mm/s]"=0.0, "Post Cut Dwell [s]"=0.0, "Ramp Time [s]"=0.0, "Start X [mm]"=0.0, "Start Y [mm]"=0.0, "Slice Length [mm]"=0.0, "Slice Axis"=enum."Y Axis", "Controller VISA Ref"="COM4"}, "Table Stages"={"X Stage"={"Position"=0.0, "Is.Enabled?"=FALSE, "Is.Connected?"=FALSE, "Device SN"="45876539", "AccelerationMaximum"=0.0, "VelocityMaximum"=0.0, "Acceleration"=0.0, "Velocity"=0.0, "waitTimeout (ms)"=0, "Model"=enum."None", "Is.Homed?"=FALSE}, "Y Stage"={"Position"=0.0, "Is.Enabled?"=FALSE, "Is.Connected?"=FALSE, "Device SN"="45876539", "AccelerationMaximum"=0.0, "VelocityMaximum"=0.0, "Acceleration"=0.0, "Velocity"=0.0, "waitTimeout (ms)"=0, "Model"=enum."None", "Is.Homed?"=FALSE}, "Z Stage"={"Position"=0.0, "Is.Enabled?"=FALSE, "Is.Connected?"=FALSE, "Device SN"="45876539", "AccelerationMaximum"=0.0, "VelocityMaximum"=0.0, "Acceleration"=0.0, "Velocity"=0.0, "waitTimeout (ms)"=0, "Model"=enum."None", "Is.Homed?"=FALSE}}, "Imaging Parameter"={"Raster Scan Direction"=enum."Bi Directional", "Pixel Dwell Time [Clock Cycles]"=1, "Flyback Time [Clock Cycles]"=0, "XY Center [um]"={"X"=1.0, "Y"=1.0}, "Pixel Step Size [um]"=1.0, "XY Image Size"=enum."256 x 256", "Custom"=FALSE, "Custom Size"={"X"=1, "Y"=1}, "Line Averages"=1}, "Galvo HW Parameters"={"Analog Out Channel"="GalvoCtrl/ao0,GalvoCtrl/ao1", "Min Voltage"=-10.0, "Max Voltage"=10.0, "Pixel Clock Source"="/GalvoCtrl/PFI0", "Sample Rate"=1000.0, "Line Clock Out Ch"="GalvoCtrl/port0/line0"}, "Alazar parameters"={"Trigger Settings"={"General Trigger Settings"={"Trigger Operation"=0, "Coupling ID"=2, "Range ID"=2, "Delay"=0, "Timeout Ticks"=0, "Mode"=1, "Parameter"=1}, "Trigger Engine 1"={"Trigger Engine"=0, "Source"=2, "Slope"=1, "Level"=140}, "Trigger Engine 2"={"Trigger Engine"=1, "Source"=3, "Slope"=1, "Level"=140}}, "Capture Clock"={"Sample Rate"=100, "Decimation"=0, "Source"=2, "Edge"=0}, "Device ID"={"System ID"=1, "Board ID"=1}, "Ch A Input Control"={"Channel"=1, "Coupling"=2, "Range"=10, "Impedance"=2}, "Ch B Input Control"={"Channel"=2, "Coupling"=2, "Range"=10, "Impedance"=2}, "Acq Settings"={"Window Type"=1, "Record Length"=1440, "Footer"=0, "Output Format"=10, "Offset"=0, "Records Per Buffer"=2048, "Samples per record"=2048, "Records Count (Records/Acq)"=2147483647}, "Cluster"={"FFT value magnification"=1000.0, "max queue size (-1, unlimited)"=-1, "File Type"=enum."Tiff", "file path"=path "C:/Users/BoasLab/Documents/Data/Alazar data/B-line/data/test.tif", "#A-lines to save"=2048, "#Z pixels to save"=2048, "ImageDescription"="", "Convert to U16?"=FALSE}}, "Mosaic Paramter"={"X Axis"={"Start [mm]"=0.0, "Steps [pts]"=0, "End [mm]"=0.0}, "Y Axis"={"Start [mm]"=0.0, "Steps [pts]"=0, "End [mm]"=0.0}, "Scan Pattern"=enum."Uni-directional", "Overlap Options"={"Overlap Type"=enum."No Overlap", "Percent Overlap"=0, "Justify"=enum."Start"}}} ("System Parameters"), "Vibratome"=w268, "Optical Parameters"=w267, "Imaging Parameter"=w266, "Galvo HW Parameters"=w265, "Alazar parameters"=w264, "Table Stages"=w263, "Mosaic Paramter"=w260) -> (w261:T30)
            n98 = local read "Save"() -> (w259:bool)
            n99 = local read "Init"() -> (w271:bool)
            n100 = call "Scan Module.vi"("Save?"=w259, "Channel"="Channel", "System Parameters [In]"=w261, "Error In"=w270, "Init"=w271) -> ("Finished?"=w269:bool, "Current Position"=→"Current Position":cluster{"X":dbl, "Y":dbl}, "Error Out"=w273:errorcluster)  [unwired: 8 in]
            n101 = local write "Init"(w269) -> ()
          }
        }
      }
      frame Error {
        n102 = local write "Error Out"(w284) -> ()
        n103 = call <vilib>:"Clear Errors.vi"("error in (no error)"=w284) -> ("error out"=w276:errorcluster)  [unwired: 5 in, 1 out]
        n104 = call "Queue Manager.vi"("Queue Name"=QueueNames."Main Scan Processor", "Action"=Queue_Manager_Actions."Flush Queue", "Error In"=w276) -> ("Error Out"=w275:errorcluster)  [unwired: 4 in, 4 out]
        n105 = call "Queue Manager.vi"("Queue Name"=QueueNames."Main Scan Processor", "timeout in ms (-1)"=-1, "Action"=Queue_Manager_Actions."Enqueue", "Error In"=w275, "Message Packet Array"=T24[] [{"Message"="Exit", "Parameter"=variant}] ("Message Packet [In]")) -> ("Error Out"=w279:errorcluster)  [unwired: 2 in, 4 out]
      }
    }
  }
  n106 = while {
    shift-right: [w286] -> w17
    shift-left: w2 -> [w285]
    stop <- w287 stop-if-true
    # "Main GUI"
    n107 = case shown="No Error" w285 {
      selector: w285 -> [w288 w519]
      tunnel: [w292 _] -> w287
      tunnel: [w289 w507] -> w286
      frame No Error {
        n108 = call "Queue Manager.vi"("Queue Name"=QueueNames."Main GUI", "Action"=Queue_Manager_Actions."Dequeue", "Error In"=w288) -> ("Error Out"=w295:errorcluster, "Message Packet [Out]"=w294:T24)  [unwired: 4 in, 3 out]
        n109 = Unbundle(w294) -> ("Message"=w290:string, "Parameter"=w293:variant)
        n110 = case shown="\"Wait for User Input\"" w290 {
          tunnel: w295 -> [w301 w332 w343 w381 w388 w402 w414 w502 w506]
          tunnel: w293 -> [_ _ _ _ _ _ _ _ _]
          tunnel: [w300 w328 w339 w363 w384 w400 w415 w503 w506] -> w289
          tunnel: [_ _ _ _ _ _ _ TRUE _] -> w292
          frame "Init" {
            n111 = call "Queue Manager.vi"("Queue Name"=QueueNames."Main GUI", "Action"=Queue_Manager_Actions."Enqueue", "Error In"=w301, "Message Packet Array"=T24[] [{"Message"="Init Variables", "Parameter"=variant}, {"Message"="Set Front Panel", "Parameter"=variant}, {"Message"="Update User Settings", "Parameter"=variant}, {"Message"="Configure Hardware", "Parameter"=variant}, {"Message"="Wait for Complete", "Parameter"=variant}, {"Message"="Wait for User Input", "Parameter"=variant}]) -> ("Error Out"=w300:errorcluster)  [unwired: 3 in, 4 out]
          }
          frame "Init Variables" {
            w311 = Queue_Manager_Actions."Init" ("Action")
            (unwired) enum32{"Scan", "Config", "Manual Contorls"}."Scan" ("Control Panel")
            n112 = call "Status Queue.vi"("Action"=Queue_Manager_Actions."Enqueue", "Error In"=w332, "Status Message [In]"="Initializing Variables...") -> ("Error Out"=w327:errorcluster)  [unwired: 7 in, 1 out]
            n113 = local write "Error Out"(errorcluster {"status"=FALSE, "code"=0, "source"=""} ("error constant")) -> ()
            n114 = control-ref of="This VI"() -> (w330:refnum<vi>)
            n115 = call "Defer Panel Updates.vi"("Action"=enum16{"Init", "Freeze", "Unfreeze"}."Init", "Error In"=w327, "reference"=w330) -> ("Error Out"=w305:errorcluster)  [unwired: 8 in]
            n116 = call "Image Queue.vi"("Action"=Queue_Manager_Actions."Init", "Error In"=w305) -> ("Error Out"=w303:errorcluster)  [unwired: 8 in, 1 out]
            n117 = call "Mosaic status.vi"("Actions"=FGV_Actions."Init", "Error In"=w303) -> ("Error Out"=w307:errorcluster)  [unwired: 7 in, 2 out]
            n118 = call "System Parameters - FGV.vi"("Actions"=FGV_Actions."Init", "Error In"=w307) -> ("Error Out"=w315:errorcluster)  [unwired: 8 in, 1 out]
            n119 = call "Data Queue2.vi"("max queue size (-1, unlimited)"=100 ("y"), "Action"=w311, "error in (no error)"=w315) -> ("error out"=w304:errorcluster)  [unwired: 5 in, 3 out]
            n120 = call "display queue.vi"("Action"=w311, "error in (no error)"=w304, "max queue size (-1, unlimited)"=100) -> ("error out"=w312:errorcluster)  [unwired: 4 in, 4 out]
            n121 = call "Trimmed data queue.vi"("max queue size (-1, unlimited)"=100, "Action"=w311, "error in (no error)"=w312) -> ("error out"=w313:errorcluster)  [unwired: 5 in, 3 out]
            n122 = disable-structure shown="Disabled" {
              disable-tunnel: [w334 w338] -> w317
              disable-tunnel: w313 -> [w333 w338]
              frame Disabled {
                n123 = call "Read Config from File.vi"("error in (no error)"=w333) -> ("error out"=w337:errorcluster, "System Parameters"=w335:T30)  [unwired: 9 in]
                n124 = call "System Parameters - FGV.vi"("Actions"=FGV_Actions."Set", "Error In"=w337, "System Parameters [In]"=w335) -> ("Error Out"=w334:errorcluster)  [unwired: 7 in, 1 out]
              }
              frame Enabled {
              }
            }
            n125 = call "FGV - Scan Status.vi"("Actions"=FGV_Actions."Init", "Error In"=w317) -> ("Error Out"=w316:errorcluster)  [unwired: 7 in, 2 out]
            n126 = control-ref of="Imaging Parameter"() -> (w320:refnum<vi>)
            n127 = call "Set Front Panel Custom Image Size Cluster Control.vi"("error in (no error)"=w316, "Enable/Disable"=FALSE, "Init"=TRUE, "Imaging Parameter"=w320) -> ("error IO"=w322:errorcluster)  [unwired: 7 in]
            n128 = call "FGV - Acquisition Status.vi"("Actions"=FGV_Actions."Init", "Error In"=w322) -> ("Error Out"=w328:errorcluster, "Scan Type [Out]"=w323:T6)  [unwired: 7 in, 1 out]
            n129 = local write "Scan Type"(w323) -> ()
          }
          frame "Set Front Panel" {
            n130 = call "Status Queue.vi"("Action"=Queue_Manager_Actions."Enqueue", "Error In"=w343, "Status Message [In]"="Setting Front Panel Controls...") -> ("Error Out"=w344:errorcluster)  [unwired: 7 in, 1 out]
            n131 = call "Defer Panel Updates.vi"("Action"=enum16{"Init", "Freeze", "Unfreeze"}."Freeze", "Error In"=w344) -> ("Error Out"=w352:errorcluster)  [unwired: 9 in]
            n132 = call "FGV - Acquisition Status.vi"("Actions"=FGV_Actions."Get", "Error In"=w352) -> ("Error Out"=w349:errorcluster, "Scan Type [Out]"=w347:T6, "Status Out"=w348:bool)  [unwired: 7 in]
            n133 = case "Acquiring?" shown="False" w348 {
              tunnel: [w356 w361] -> w350
              tunnel: w349 -> [w357 w361]
              tunnel: w347 -> [w355 _]
              frame False {
                # "Non-Acquiring FP States"
                n134 = disable-structure shown="Enabled" {
                  disable-tunnel: w357 -> [w360 _]
                  disable-tunnel: [w359 _] -> w356
                  disable-tunnel: w355 -> [w358 _]
                  frame Disabled {
                    n135 = call "Set Main GUI for Different Acquire States.vi"("Error In"=w360, "Scan Type"=w358) -> ("Error Out"=w359:errorcluster)  [unwired: 9 in]
                  }
                  frame Enabled {
                  }
                }
              }
              frame True {
                # "Acquiring FP States"
              }
            }
            n136 = call "Defer Panel Updates.vi"("Action"=enum16{"Init", "Freeze", "Unfreeze"}."Unfreeze", "Error In"=w350) -> ("Error Out"=w340:errorcluster)  [unwired: 9 in]
            n137 = call "Status Queue.vi"("Action"=Queue_Manager_Actions."Enqueue", "Error In"=w340, "Status Message [In]"="Finished Setting Front Panel.") -> ("Error Out"=w339:errorcluster)  [unwired: 7 in, 1 out]
          }
          frame "Update User Settings" {
            n138 = disable-structure shown="Enabled" {
              disable-tunnel: [_ Queue_Manager_Actions."Enqueue" ("Action")] -> w375
              frame Disabled {
                n139 = local read "Vibratome"() -> ()  [unwired: 1 in]
                n140 = local read "Imaging Parameter"() -> ()  [unwired: 1 in]
                n141 = local read "Optical Parameters"() -> ()  [unwired: 1 in]
              }
              frame Enabled {
              }
            }
            n142 = call "Status Queue.vi"("Action"=w375, "Error In"=w381, "Status Message [In]"="Loading User Settings...") -> ("Error Out"=w379:errorcluster)  [unwired: 7 in, 1 out]
            n143 = call "Defer Panel Updates.vi"("Action"=enum16{"Init", "Freeze", "Unfreeze"}."Freeze", "Error In"=w379) -> ("Error Out"=w374:errorcluster)  [unwired: 9 in]
            n144 = call "Set Front Panel Custom Image Size Cluster Control.vi"("error in (no error)"=w374, "Enable/Disable"=TRUE) -> ("error IO"=w377:errorcluster)  [unwired: 9 in]
            n145 = call "Defer Panel Updates.vi"("Action"=enum16{"Init", "Freeze", "Unfreeze"}."Unfreeze", "Error In"=w377) -> ("Error Out"=w364:errorcluster)  [unwired: 9 in]
            n146 = Bundle By Name(cluster=T30 {"Optical Parameters"={"Obj. Focal Length [mm]"=0.0, "Scan Lens EFL[mm]"=0.0, "Tube Lens EFL[mm]"=0.0, "Galvo V Range (+/-)"=0.0, "Galvo Max Half Angle [Deg]"=0.0, "Max Galvo Range[%]"=0.0}, "Vibratome"={"Z Bottom [mm]"=0.0, "Pre Cut Dwell [s]"=0.0, "Blade Frequency [RPM]"=0, "Slice Speed [mm/s]"=0.0, "Post Cut Dwell [s]"=0.0, "Ramp Time [s]"=0.0, "Start X [mm]"=0.0, "Start Y [mm]"=0.0, "Slice Length [mm]"=0.0, "Slice Axis"=enum."Y Axis", "Controller VISA Ref"="COM4"}, "Table Stages"={"X Stage"={"Position"=0.0, "Is.Enabled?"=FALSE, "Is.Connected?"=FALSE, "Device SN"="45876539", "AccelerationMaximum"=0.0, "VelocityMaximum"=0.0, "Acceleration"=0.0, "Velocity"=0.0, "waitTimeout (ms)"=0, "Model"=enum."None", "Is.Homed?"=FALSE}, "Y Stage"={"Position"=0.0, "Is.Enabled?"=FALSE, "Is.Connected?"=FALSE, "Device SN"="45876539", "AccelerationMaximum"=0.0, "VelocityMaximum"=0.0, "Acceleration"=0.0, "Velocity"=0.0, "waitTimeout (ms)"=0, "Model"=enum."None", "Is.Homed?"=FALSE}, "Z Stage"={"Position"=0.0, "Is.Enabled?"=FALSE, "Is.Connected?"=FALSE, "Device SN"="45876539", "AccelerationMaximum"=0.0, "VelocityMaximum"=0.0, "Acceleration"=0.0, "Velocity"=0.0, "waitTimeout (ms)"=0, "Model"=enum."None", "Is.Homed?"=FALSE}}, "Imaging Parameter"={"Raster Scan Direction"=enum."Bi Directional", "Pixel Dwell Time [Clock Cycles]"=1, "Flyback Time [Clock Cycles]"=0, "XY Center [um]"={"X"=1.0, "Y"=1.0}, "Pixel Step Size [um]"=1.0, "XY Image Size"=enum."256 x 256", "Custom"=FALSE, "Custom Size"={"X"=1, "Y"=1}, "Line Averages"=1}, "Galvo HW Parameters"={"Analog Out Channel"="GalvoCtrl/ao0,GalvoCtrl/ao1", "Min Voltage"=-10.0, "Max Voltage"=10.0, "Pixel Clock Source"="/GalvoCtrl/PFI0", "Sample Rate"=1000.0, "Line Clock Out Ch"="GalvoCtrl/port0/line0"}, "Alazar parameters"={"Trigger Settings"={"General Trigger Settings"={"Trigger Operation"=0, "Coupling ID"=2, "Range ID"=2, "Delay"=0, "Timeout Ticks"=0, "Mode"=1, "Parameter"=1}, "Trigger Engine 1"={"Trigger Engine"=0, "Source"=2, "Slope"=1, "Level"=140}, "Trigger Engine 2"={"Trigger Engine"=1, "Source"=3, "Slope"=1, "Level"=140}}, "Capture Clock"={"Sample Rate"=100, "Decimation"=0, "Source"=2, "Edge"=0}, "Device ID"={"System ID"=1, "Board ID"=1}, "Ch A Input Control"={"Channel"=1, "Coupling"=2, "Range"=10, "Impedance"=2}, "Ch B Input Control"={"Channel"=2, "Coupling"=2, "Range"=10, "Impedance"=2}, "Acq Settings"={"Window Type"=1, "Record Length"=1440, "Footer"=0, "Output Format"=10, "Offset"=0, "Records Per Buffer"=2048, "Samples per record"=2048, "Records Count (Records/Acq)"=2147483647}, "Cluster"={"FFT value magnification"=1000.0, "max queue size (-1, unlimited)"=-1, "File Type"=enum."Tiff", "file path"=path "C:/Users/BoasLab/Documents/Data/Alazar data/B-line/data/test.tif", "#A-lines to save"=2048, "#Z pixels to save"=2048, "ImageDescription"="", "Convert to U16?"=FALSE}}, "Mosaic Paramter"={"X Axis"={"Start [mm]"=0.0, "Steps [pts]"=0, "End [mm]"=0.0}, "Y Axis"={"Start [mm]"=0.0, "Steps [pts]"=0, "End [mm]"=0.0}, "Scan Pattern"=enum."Uni-directional", "Overlap Options"={"Overlap Type"=enum."No Overlap", "Percent Overlap"=0, "Justify"=enum."Start"}}} ("System Parameters"), "Vibratome"="Vibratome", "Optical Parameters"="Optical Parameters", "Imaging Parameter"="Imaging Parameter", "Galvo HW Parameters"="Galvo HW Parameters", "Alazar parameters"="Alazar parameters", "Table Stages"="Table Stages", "Mosaic Paramter"="Mosaic Paramter") -> (w370:T30)
            n147 = call "System Parameters - FGV.vi"("Actions"=FGV_Actions."Set", "Error In"=w364, "System Parameters [In]"=w370) -> ("Error Out"=w363:errorcluster)  [unwired: 7 in, 1 out]
          }
          frame "Configure Hardware" {
            n148 = call "Status Queue.vi"("Action"=Queue_Manager_Actions."Enqueue", "Error In"=w388, "Status Message [In]"="Initializing Hardware...") -> ("Error Out"=w387:errorcluster)  [unwired: 7 in, 1 out]
            n149 = Build Array(T24 {"Message"="Init Hardware", "Parameter"=variant} ("Message Packet [In]")) -> (w385:T24[])
            n150 = call "Queue Manager.vi"("Queue Name"=QueueNames."Main Scan Processor", "Action"=Queue_Manager_Actions."Enqueue", "Error In"=w387, "Message Packet Array"=w385) -> ("Error Out"=w384:errorcluster)  [unwired: 3 in, 4 out]
          }
          frame "Wait for Complete" {
            n151 = call "TickTock.vi"("Error In"=w402) -> ("Error Out"=w398:errorcluster, "Current Time (Out)"=w397:timestamp)  [unwired: 8 in, 1 out]
            n152 = while {
              shift-right: [w405] -> w399
              shift-left: w398 -> [w413]
              tunnel: w397 -> [w412]
              tunnel: [w403] -> w396
              stop <- w404 stop-if-true
              n153 = call "Inline Wait.vi"("Error In"=w413, "milliseconds to wait"=u32 100) -> ("Error Out"=w409:errorcluster)  [unwired: 9 in]
              n154 = call "TickTock.vi"("Error In"=w409, "Current Time (In)"=w412) -> ("Error Out"=w405:errorcluster, "dt"=w411:dbl)  [unwired: 7 in, 1 out]
              n155 = Greater?(x=60000.0, y=w411) -> (0:w403:bool)
              n156 = global read "Main Scan Processor Status.vi" "Busy"() -> (w407:bool)
              n157 = Not(x=w407) -> (.not. x?=w406:bool)
              n158 = Or(x=w403, y=w406) -> (x .or. y?=w404:bool)
            }
            n159 = Select(t="Completed." ("Status Message [In]"), s=w396, f="Operation timed out." ("Status Message [In]")) -> (s? t:f=w393:string)
            n160 = call "Status Queue.vi"("Action"=Queue_Manager_Actions."Enqueue", "Error In"=w399, "Status Message [In]"=w393) -> ("Error Out"=w400:errorcluster)  [unwired: 7 in, 1 out]
          }
          frame "Wait for User Input" {
            n161 = event shown="[5] \"Acquire\": Value Change" {
              selector: _ -> [_ _ _ _ _ _]
              dyn-events: _ -> [_ _ _ _ _ _]
              timeout: _ -> [_ _ _ _ _ _]
              tunnel: [w416 w428 w445 w461 w473 w489] -> w415
              tunnel: w414 -> [w416 w419 w447 w458 w477 w491]
              event Timeout {
                n162 = event-data() -> ()  [unwired: 1 in, 3 out]
              }
              event "Quit": Value Change {
                n163 = event-data() -> ()  [unwired: 1 in, 1 out]
                n164 = flat-sequence {
                  tunnel: w419 -> [w430]
                  tunnel: [w433] -> w417
                  tunnel: [w439] -> w418
                  tunnel: w417 -> [w439]
                  frame #0 {
                    n165 = call "FGV - Acquisition Status.vi"("Actions"=FGV_Actions."Set", "Error In"=w430, "Status In"=FALSE) -> ("Error Out"=w429:errorcluster)  [unwired: 6 in, 2 out]
                    n166 = call "Queue Manager.vi"("Queue Name"=QueueNames."Main Saving", "timeout in ms (-1)"=-1, "Action"=Queue_Manager_Actions."Enqueue", "Error In"=w429, "Message Packet Array"=T24[] [{"Message"="Close", "Parameter"=variant}] ("Message Packet [In]")) -> ("Error Out"=w433:errorcluster)  [unwired: 2 in, 4 out]
                  }
                  frame #1 {
                    n167 = Wait (ms)(milliseconds to wait=u32 10) -> ()  [unwired: 1 out]
                  }
                }
                n168 = call "Status Queue.vi"("Action"=Queue_Manager_Actions."Enqueue", "Error In"=w418, "Status Message [In]"="Exiting Software...") -> ("Error Out"=w422:errorcluster)  [unwired: 7 in, 1 out]
                n169 = call "Set Main GUI for Different Acquire States.vi"("Error In"=w422, "Scan Type"=ScanType."Single Frame" ("Scan Type [Out]")) -> ("Error Out"=w421:errorcluster)  [unwired: 9 in]
                n170 = Build Array(T24 {"Message"="Exit", "Parameter"=variant} ("Message Packet [In]")) -> (w425:T24[])
                n171 = call "Queue Manager.vi"("Action"=Queue_Manager_Actions."Enqueue All", "Error In"=w421, "Message Packet Array"=w425) -> ("Error Out"=w428:errorcluster)  [unwired: 4 in, 4 out]
              }
              event "Image": Value Change {
                w448 = 2 items=["No Event"=0, "Click Event"=1, "Draw Event"=2, "Size Event"=4, "Scroll Event"=5, "Double Click Event"=8]
                n172 = event-data() -> ("CtlRef"=w440:refnum<vi>)  [unwired: 1 in, 5 out]
                n173 = Build Array(w448) -> (w449:i32[])
                n174 = invoke class="ImageControl" method="Get Last Event"(reference=w440, error in=w447, "Which Events"=w449) -> (error out=w446:errorcluster)  [unwired: 5 in, 7 out]
                n175 = Build Array(T24 {"Message"="Wait for User Input", "Parameter"=variant} ("Message Packet [In]")) -> (w441:T24[])
                n176 = call "Queue Manager.vi"("Queue Name"=QueueNames."Main GUI", "Action"=Queue_Manager_Actions."Enqueue", "Error In"=w446, "Message Packet Array"=w441) -> ("Error Out"=w445:errorcluster)  [unwired: 3 in, 4 out]
              }
              event Value Change {
                n177 = event-data() -> ("NewVal"=w453:T31)  [unwired: 1 in]
                n178 = Add(x=w453, y=5) -> (x+y=w467:i32)
                n179 = Power Of 2(x=w467) -> (2^x=w466:dbl)
                n180 = call "System Parameters - FGV.vi"("Actions"=FGV_Actions."Get", "Error In"=w458) -> ("Error Out"=w457:errorcluster, "System Parameters"=w455:T30)  [unwired: 8 in]
                n181 = Bundle By Name(cluster=w455, "Imaging Parameter.XY Image Size"=w453) -> (w454:T30)
                n182 = local read "Imaging Parameter"() -> (w452:T4)
                n183 = To Unsigned Word Integer(number=w466) -> (unsigned 16bit integer=w450:u16)
                n184 = Bundle By Name(cluster=w452, "Custom Size.X"=w450, "Custom Size.Y"=w450) -> (w451:T4)
                n185 = local write "Imaging Parameter"(w451) -> ()
                n186 = call "System Parameters - FGV.vi"("Actions"=FGV_Actions."Set", "Error In"=w457, "System Parameters [In]"=w454) -> ("Error Out"=w456:errorcluster)  [unwired: 7 in, 1 out]
                n187 = Build Array(T24 {"Message"="Wait for User Input", "Parameter"=variant} ("Message Packet [In]")) -> (w462:T24[])
                n188 = call "Queue Manager.vi"("Queue Name"=QueueNames."Main GUI", "Action"=Queue_Manager_Actions."Enqueue", "Error In"=w456, "Message Packet Array"=w462) -> ("Error Out"=w461:errorcluster)  [unwired: 3 in, 4 out]
              }
              event Value Change {
                n189 = event-data() -> ()  [unwired: 1 in, 6 out]
                n190 = call "FGV - Acquisition Status.vi"("Actions"=FGV_Actions."Get") -> ("Status Out"=w472:bool)  [unwired: 8 in, 2 out]
                n191 = call "FGV - Acquisition Status.vi"("Actions"=FGV_Actions."Set", "Scan Type [In]"="Scan Type", "Status In"=w472) -> ()  [unwired: 6 in, 3 out]
                n192 = call "Queue Manager.vi"("Queue Name"=QueueNames."Main GUI", "Action"=Queue_Manager_Actions."Enqueue", "Error In"=w477, "Message Packet Array"=T24[] [{"Message"="Set Front Panel", "Parameter"=variant}, {"Message"="Wait for User Input", "Parameter"=variant}]) -> ("Error Out"=w473:errorcluster)  [unwired: 3 in, 4 out]
              }
              event "Acquire": Value Change {
                w488 = Queue_Manager_Actions."Enqueue" ("Action")
                n193 = event-data() -> ()  [unwired: 1 in, 6 out]
                n194 = local write "Init"(TRUE) -> ()
                n195 = call "Queue Manager.vi"("Queue Name"=QueueNames."Main GUI", "Action"=w488, "Error In"=w491, "Message Packet Array"=T24[] [{"Message"="Wait for User Input", "Parameter"=variant}]) -> ("Error Out"=w490:errorcluster)  [unwired: 3 in, 4 out]
                n196 = call "FGV - Acquisition Status.vi"("Actions"=FGV_Actions."Get") -> ("Status Out"=w482:bool)  [unwired: 8 in, 2 out]
                n197 = case "Start Acquisition?" shown="False" w482 {
                  tunnel: w490 -> [w492 w498]
                  tunnel: [w497 w498] -> w489
                  tunnel: w488 -> [w496 _]
                  frame False {
                    # "Starts Acquisition if Current Acquisition Status is \"Off\""
                    n198 = Build Array(T24 {"Message"="Acquire", "Parameter"=variant} ("Message Packet [In]")) -> (w493:T24[])
                    n199 = call "Queue Manager.vi"("Queue Name"=QueueNames."Main Scan Processor", "Action"=w496, "Error In"=w492, "Message Packet Array"=w493) -> ("Error Out"=w497:errorcluster)  [unwired: 3 in, 4 out]
                  }
                  frame True {
                    # "Stops Acquisition if Current Status is On"
                  }
                }
                n200 = Not(x=w482) -> (.not. x?=w483:bool)
                n201 = call "FGV - Acquisition Status.vi"("Actions"=FGV_Actions."Get") -> ("Error Out"=w481:errorcluster, "Scan Type [Out]"=w479:T6)  [unwired: 8 in, 1 out]
                n202 = call "FGV - Acquisition Status.vi"("Actions"=FGV_Actions."Set", "Error In"=w481, "Scan Type [In]"=w479, "Status In"=w483) -> ()  [unwired: 5 in, 3 out]
              }
            }
          }
          frame "Exit" {
            n203 = disable-structure shown="Disabled" {
              frame Disabled {
                w505 = enum16{"open", "save", "close"}."close" ("Action")
                n204 = call "Save text module - Copy (2).vi"("Action"=w505) -> ()  [unwired: 11 in]
                n205 = call "Save text module - Copy.vi"("Action"=w505) -> ()  [unwired: 11 in]
                n206 = call "Save text module.vi"("Action"=w505) -> ()  [unwired: 11 in]
              }
              frame Enabled {
              }
            }
            n207 = call "System Parameters - FGV.vi"("Actions"=FGV_Actions."Get", "Error In"=w502) -> ("Error Out"=w501:errorcluster, "System Parameters"=w499:T30)  [unwired: 8 in]
            n208 = call "Write Config to File.vi"("error in (no error)"=w501, "System Parameters"=w499) -> ("error out"=w503:errorcluster)  [unwired: 9 in]
          }
          frame Default {
          }
        }
      }
      frame Error {
        n209 = call <vilib>:"Clear Errors.vi"("error in (no error)"=w519) -> ("error out"=w508:errorcluster)  [unwired: 5 in, 1 out]
        n210 = local write "Error Out"(w519) -> ()
        n211 = flat-sequence {
          tunnel: w508 -> [w521]
          tunnel: [w520] -> w518
          tunnel: [w527] -> w509
          tunnel: w518 -> [w527]
          frame #0 {
            n212 = call "Queue Manager.vi"("Queue Name"=QueueNames."Main Saving", "timeout in ms (-1)"=-1, "Action"=Queue_Manager_Actions."Enqueue", "Error In"=w521, "Message Packet Array"=T24[] [{"Message"="Close", "Parameter"=variant}] ("Message Packet [In]")) -> ("Error Out"=w520:errorcluster)  [unwired: 2 in, 4 out]
          }
          frame #1 {
            n213 = Wait (ms)(milliseconds to wait=u32 10) -> ()  [unwired: 1 out]
          }
        }
        n214 = call "Status Queue.vi"("Action"=Queue_Manager_Actions."Enqueue", "Error In"=w509, "Status Message [In]"="Exiting Software...") -> ("Error Out"=w512:errorcluster)  [unwired: 7 in, 1 out]
        n215 = call "Set Main GUI for Different Acquire States.vi"("Error In"=w512, "Scan Type"=ScanType."Single Frame" ("Scan Type [Out]")) -> ("Error Out"=w511:errorcluster)  [unwired: 9 in]
        n216 = Build Array(T24 {"Message"="Exit", "Parameter"=variant} ("Message Packet [In]")) -> (w515:T24[])
        n217 = call "Queue Manager.vi"("Action"=Queue_Manager_Actions."Enqueue All", "Error In"=w511, "Message Packet Array"=w515) -> ("Error Out"=w507:errorcluster)  [unwired: 4 in, 4 out]
      }
    }
  }
  n218 = call "Queue Manager.vi"("Queue Name"=QueueNames."Main Processing", "Action"=Queue_Manager_Actions."Release Queue", "Error In"=w3) -> ()  [unwired: 4 in, 5 out]
  n219 = call "Queue Manager.vi"("Queue Name"=QueueNames."Main Display", "Action"=Queue_Manager_Actions."Release Queue", "Error In"=w10) -> ()  [unwired: 4 in, 5 out]
  n220 = call "Queue Manager.vi"("Queue Name"=QueueNames."Main Saving", "Action"=Queue_Manager_Actions."Release Queue", "Error In"=w6) -> ()  [unwired: 4 in, 5 out]
  n221 = call "Queue Manager.vi"("Queue Name"=QueueNames."Main Scan Processor", "Action"=Queue_Manager_Actions."Release Queue", "Error In"=w12) -> ()  [unwired: 4 in, 5 out]
  n222 = call "Queue Manager.vi"("Queue Name"=QueueNames."Main GUI", "Action"=Queue_Manager_Actions."Release Queue", "Error In"=w17) -> ()  [unwired: 4 in, 5 out]
